vi "Helm Adjust Headings for PID TEST.vi"(8 "error in (no error)":errorcluster) -> (0 "error out":errorcluster)   [LabVIEW 2015]
panel:
  out "x-y":dbl
  out "Dadj":dbl
  out "Aadj":dbl
  in  "Gauge":cluster{dbl, dbl}(knob)={0.0, 16.871828399534785} scale=0.0..360.0
  # "Green Actual"
  # "Red Desirec"
  # "Negative means port turn"
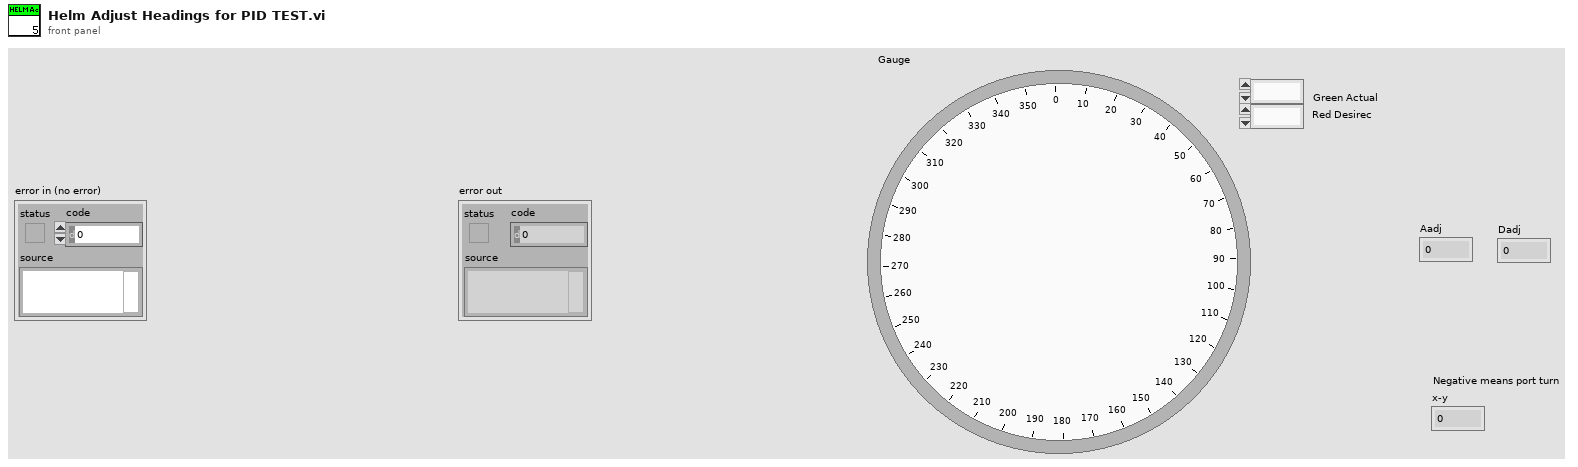
[diagram p1: front panel]
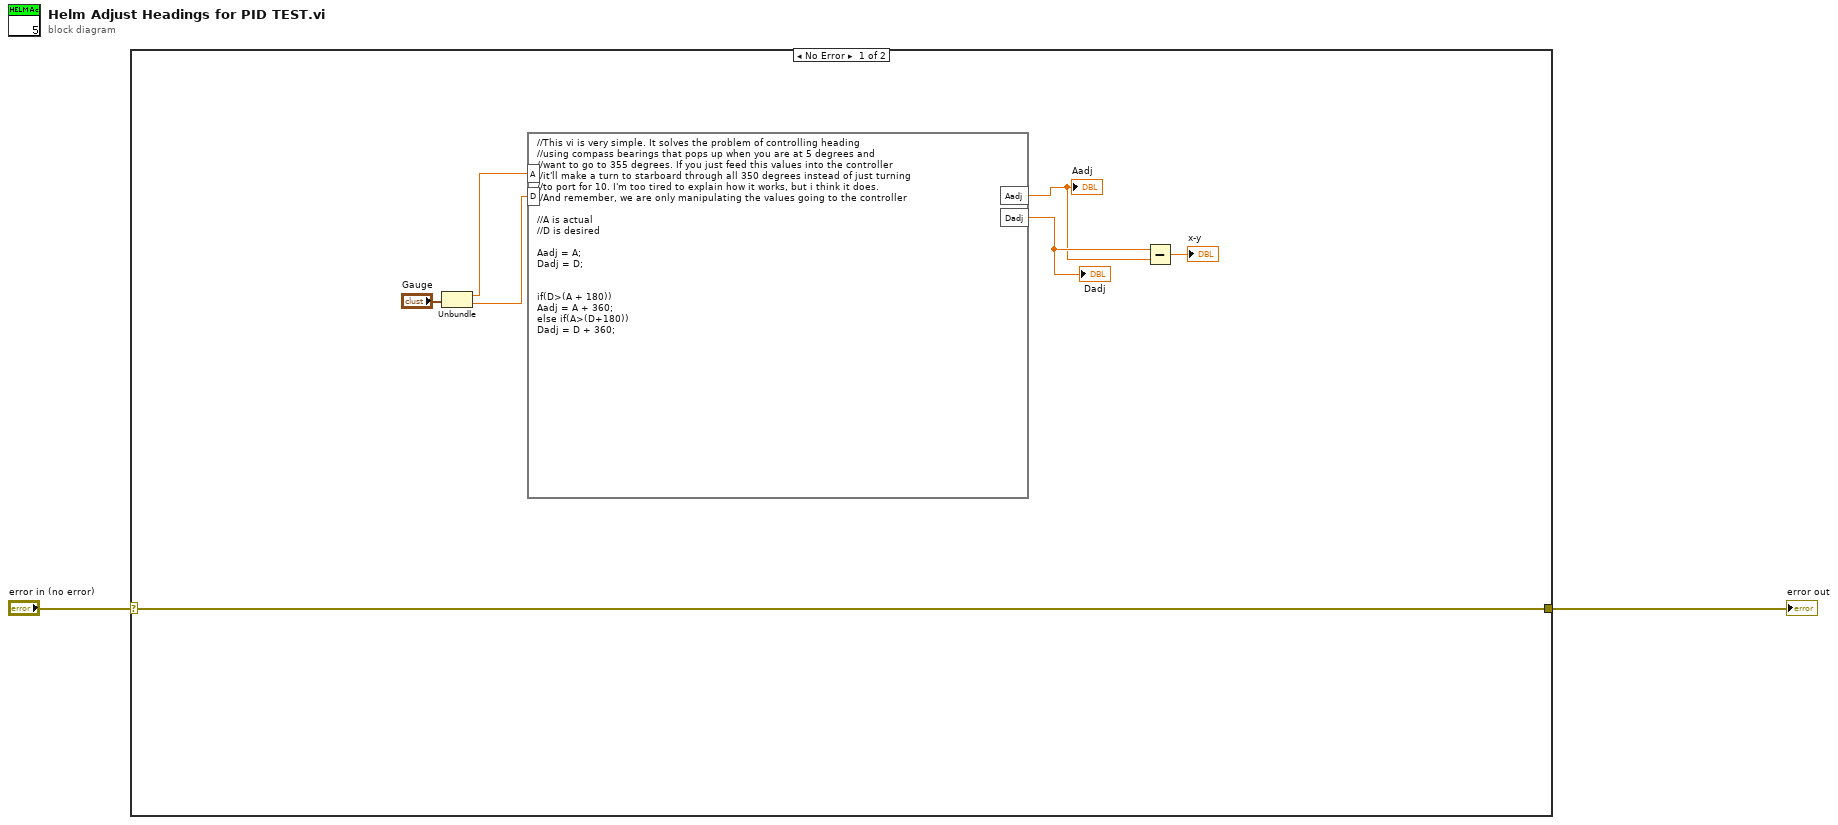
[diagram p0: block diagram]
diagram:
  n1 = case shown="No Error" "error in (no error)" {
    selector: "error in (no error)" -> [w9 w10]
    tunnel: [w9 w10] -> w1
    frame No Error {
      n2 = Unbundle("Gauge") -> (w4:dbl, w3:dbl)
      n3 = formula code="//This vi is very simple. It solves the problem of controlling heading\n//using compass bearings that pops up when you are at 5 degrees and\n//want to go to 355 degrees. If you just feed this values into the controller\n//it'll make a turn to starboard through all 350 degrees instead of just turning\n//to port for 10. I'm too tired to explain how it works, but i think it does.\n//And remember, we are only manipulating the values going to the controller\n\n//A is actual\n//D is desired\n\nAadj = A;\nDadj = D;\n\n\nif(D>(A + 180))\nAadj = A + 360;\nelse if(A>(D+180))\nDadj = D + 360;"("A"=w4, "D"=w3) -> ("Aadj"=w7:dbl, "Dadj"=w8:dbl)
      "Aadj" <- w7
      "Dadj" <- w8
      n4 = Subtract(x=w8, y=w7) -> (x-y=→"x-y":dbl)
    }
    frame Error {
    }
  }
  "error out" <- w1
